vi "Actor Core.vi"(8 "error in":errorcluster, 11 "WebSocket Actor in":refnum<class "WebSocket Server.lvclass">) -> (0 "error out":errorcluster, 3 "Actor out":refnum<class "Actor.lvclass">)   [LabVIEW 2016, in "WebSocket Actor.lvlib" / "WebSocket Server.lvclass"]
doc: "(<B>Filename</B>: Actor Framework.lvlib:Actor.lvclass:Actor Core.vi)\n\nReceives messages to the actor, reacts to them, and initiates any error handling that may shut the actor down.\n\nDescendant classes may override this VI to append parallel tasks for the actor to complete while it handles messages. Overrides use the Call Parent Method node."
uses:
  WebSocket Server.lvclass
  C:/Program Files (x86)/National Instruments/LabVIEW 2016/vi.lib/ActorFramework/Actor/Actor.lvclass
  <vilib>/ActorFramework/Actor/Actor.lvclass
  <vilib>/ActorFramework/Actor/Actor.lvclass/Actor.ctl
  <vilib>/ActorFramework/Message Enqueuer/Message Enqueuer.lvclass/Message Enqueuer.ctl
  WebSocket Server.lvclass/WebSocket Server.ctl
  <vilib>/GPower/Error/Library/Filter/FilterSingle.vi
  <vilib>/ActorFramework/Message Enqueuer/Init from Existing Queue.vi
  <vilib>/GPower/Error/Library/SplitAppended.vi
  <vilib>/GPower/Error/Library/SubVIs/ExplanationToError.vi
  <vilib>/dlg_ctls.llb/Space Constant.vi
  <vilib>/Utility/error.llb/Error Cluster From Error Code.vi
  <vilib>/Utility/error.llb/Trim Whitespace.vi
  <vilib>/Utility/error.llb/Error Code Database.vi
  <vilib>/GPower/Error/Library/Append/AppendSingle.vi
  <vilib>/ActorFramework/Message Enqueuer/Message Enqueuer.lvclass
  <vilib>/ErrorRing/Error Ring.xnode
  WebSocket Server Messages/Write listener ID Msg/Write listener ID Msg.lvclass
  WebSocket Server Messages/Add Client to Service Msg/Add Client to Service Msg.lvclass
  <vilib>/GPower/Error/GPError.lvlib
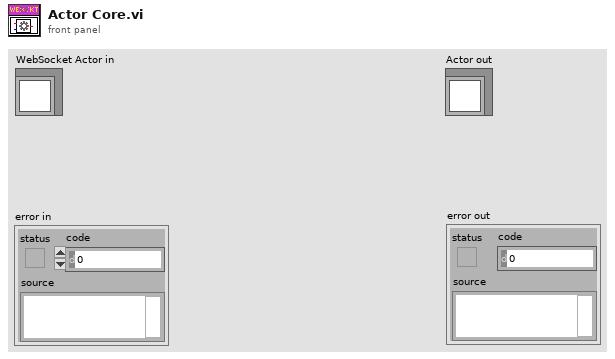
[diagram p1: front panel]
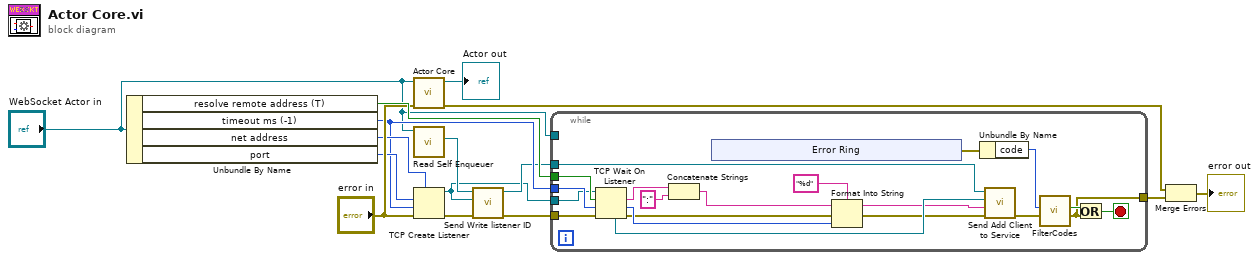
[diagram p0: block diagram]
diagram:
  n1 = Unbundle By Name("WebSocket Actor in") -> ("resolve remote address (T)"=w13:bool, "timeout ms (-1)"=w9:i32, "net address"=w10:u32, "port"=w11:u16)
  n2 = call-parent "Actor Core.vi"("error in"="error in", "Actor in"="WebSocket Actor in") -> ("error out"=w15:errorcluster, "Actor out"=→"Actor out":refnum<class "Actor.lvclass">)  [unwired: 8 in]
  n3 = call <vilib>:"Read Self Enqueuer.vi"("Actor"="WebSocket Actor in") -> ("Self Enqueuer"=w7:refnum<class "Message Enqueuer.lvclass">)  [unwired: 10 in]
  n4 = TCP Create Listener(7:w10, 8:"error in", 9:w9, 10:w11) -> (0:w8:errorcluster, 3:w3:refnum<k5>)  [unwired: 1 in, 1 out]
  n5 = call "Send Write listener ID.vi"("error in (no error)"=w8, "listener ID"=w3, "Message Enqueuer in"=w7) -> ("error out"=w4:errorcluster, "Message Enqueuer out"=w5:refnum<class "Message Enqueuer.lvclass">)  [unwired: 7 in]
  n6 = while {
    tunnel: w13 -> [w30]
    tunnel: w9 -> [w32]
    tunnel: "WebSocket Actor in" -> [_]
    tunnel: w5 -> [w29]
    tunnel: w4 -> [w28]
    tunnel: w3 -> [w27]
    tunnel: [w16] -> w1
    stop <- w18 stop-if-true
    n7 = TCP Wait On Listener(8:w28, 9:w32, 10:w30, 11:w27) -> (0:w22:errorcluster, 1:w25:u16, 2:w26:string, 4:w31:refnum<k5>)  [unwired: 1 out]
    n8 = Concatenate Strings(w26, ":" ("string")) -> (w23:string)
    n9 = xnode "Error Ring"() -> ("error out"=w35:errorcluster)
    n10 = Format Into String(format string="%d", initial string=w23, error in=w22, w25) -> (resulting string=w20:string, error out=w21:errorcluster)
    n11 = Unbundle By Name(w35) -> ("code"=w33:i32)
    n12 = call "Send Add Client to Service.vi"("error in (no error)"=w21, "Client ID"=w20, "WebSocket Connection in"=w31, "Message Enqueuer in"=w29) -> ("error out"=w34:errorcluster)  [unwired: 6 in, 1 out]
    n13 = call-poly <vilib>:"FilterCodes.vi"("Error in"=w34, "Code to filter"=w33) -> ("Error out"=w16:errorcluster, "Code filtered?"=w17:bool)  [unwired: 8 in]
    n14 = Or(x=w17, y=w16) -> (x .or. y?=w18:bool)
  }
  n15 = Merge Errors(w15, w1) -> (→"error out":errorcluster)
